vi "DSF.Engine.Framework.Initialize.Builders.vi"(8 "error in (no error)":errorcluster, 11 "Framework in":refnum<class "Framework.lvclass">) -> (0 "error out":errorcluster, 3 "Framework out":refnum<class "Framework.lvclass">)   [LabVIEW 2016, in "DSF.Engine.lvlib" / "Framework.lvclass"]
uses:
  Framework.lvclass
  Hardware/DSF.Engine.Hardware Info.lvclass
  Hardware/DSF.Engine.Hardware Info.CPU.lvclass
  BuilderManager/DSF.Engine.BuilderManager.lvclass
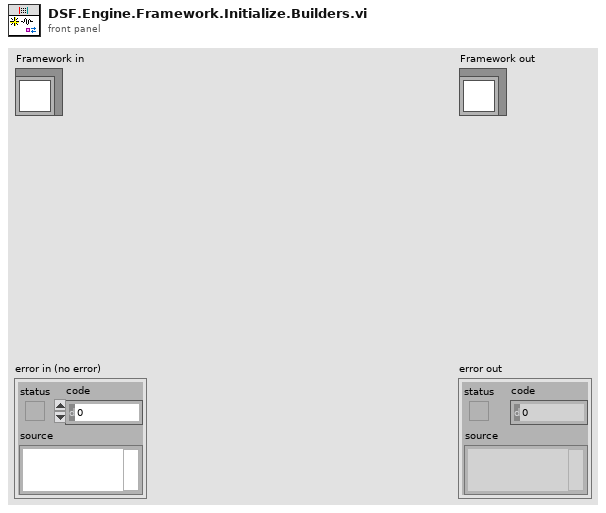
[diagram p1: front panel]
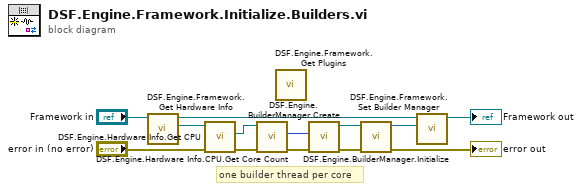
[diagram p0: block diagram]
diagram:
  # "one builder thread per core"
  n1 = call "DSF.Engine.Framework.Get Hardware Info.vi"("Framework in"="Framework in") -> ("Hardware Info"=w6:refnum<class "DSF.Engine.Hardware Info.lvclass">, "Framework out"=w4:refnum<class "Framework.lvclass">)  [unwired: 9 in]
  n2 = call "DSF.Engine.Hardware Info.Get CPU.vi"("error in (no error)"="error in (no error)", "Hardware Info in"=w6) -> ("error out"=w12:errorcluster, "CPU Info"=w13:refnum<class "DSF.Engine.Hardware Info.CPU.lvclass">)  [unwired: 7 in, 1 out]
  n3 = call "DSF.Engine.Hardware Info.CPU.Get Core Count.vi"("error in (no error)"=w12, "CPU Info in"=w13) -> ("error out"=w10:errorcluster, "Core Count"=w11:i32)  [unwired: 7 in, 1 out]
  n4 = call "DSF.Engine.Framework.Get Plugins.vi"() -> ()  [unwired: 10 in, 2 out]
  n5 = call "DSF.Engine.BuilderManager.Create.vi"("error in (no error)"=w10, "number of builders"=w11) -> ("error out"=w8:errorcluster, "Builder Manager"=w9:refnum<class "DSF.Engine.BuilderManager.lvclass">)  [unwired: 8 in]
  n6 = call "DSF.Engine.BuilderManager.Initialize.vi"("error in (no error)"=w8, "Builder Manager in"=w9) -> ("error out"=→"error out":errorcluster, "Builder Manager out"=w3:refnum<class "DSF.Engine.BuilderManager.lvclass">)  [unwired: 8 in]
  n7 = call "DSF.Engine.Framework.Set Builder Manager.vi"("Builder Manager"=w3, "Framework in"=w4) -> ("Framework out"=→"Framework out":refnum<class "Framework.lvclass">)  [unwired: 9 in]
